vi "AlazarConfigureAuxIO.vi"(3 "error in (no error)":errorcluster, 4 "Parameter":u32, 5 "Mode":u32, 6 "Handle":u32) -> (0 "error out":errorcluster, 1 "Return Code":u32, 2 "Handle":u32)   [LabVIEW 2021]
doc: "Configure the AUX I/O connector as an input or output signal."
uses:
  ATSApi.dll
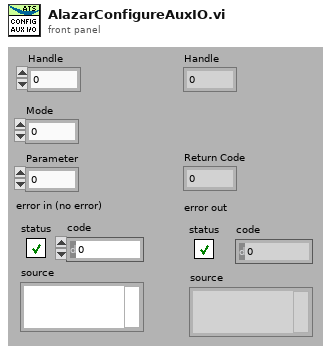
[diagram p1: front panel]
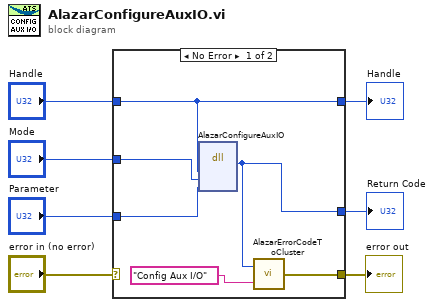
[diagram p0: block diagram]
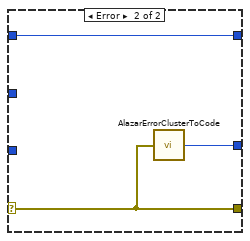
[diagram p2: hidden frame]
diagram:
  n1 = case shown="No Error" "error in (no error)" {
    selector: "error in (no error)" -> [_ w16]
    tunnel: [w9 w16] -> w6
    tunnel: [w10 w15] -> w5
    tunnel: "Handle" -> [w11 w14]
    tunnel: [w11 w14] -> w3
    tunnel: "Mode" -> [w13 _]
    tunnel: "Parameter" -> [w12 _]
    frame No Error {
      n2 = dll-call lib="ATSApi.dll" fn="AlazarConfigureAuxIO"("handle"=w11, "mode"=w13, "parameter"=w12) -> (w10:u32)  [unwired: 6 in, 2 out]
      n3 = call "AlazarErrorCodeToCluster.vi"("Message"="Config Aux I/O", "Error Code"=w10) -> ("error out"=w9:errorcluster)
    }
    frame Error {
      n4 = call "AlazarErrorClusterToCode.vi"("error in (no error)"=w16) -> ("Error Code"=w15:u32)
    }
  }
  "Handle" <- w3
  "error out" <- w6
  "Return Code" <- w5
